vi "Get Grouped Channel Settings.vi"(9 "Type":T2(ring), 10 "Group Name":string, 11 "Group Settings":T3[](array[typedef])) -> (1 "found?":bool, 2 "Channel Settings":T1[](array[typedef]), 3 "Name based Group Settings":T3[](array[typedef]))   [LabVIEW 2026, in "SystemMonitor Engine.lvlib" / "SystemMonitor Engine.lvclass"]
uses:
  SystemMonitor Engine.lvclass
  Shared/GroupSettings.ctl
  Shared/GroupedChannel.ctl
  SystemMonitor Engine.lvclass/SystemMonitor Engine.ctl
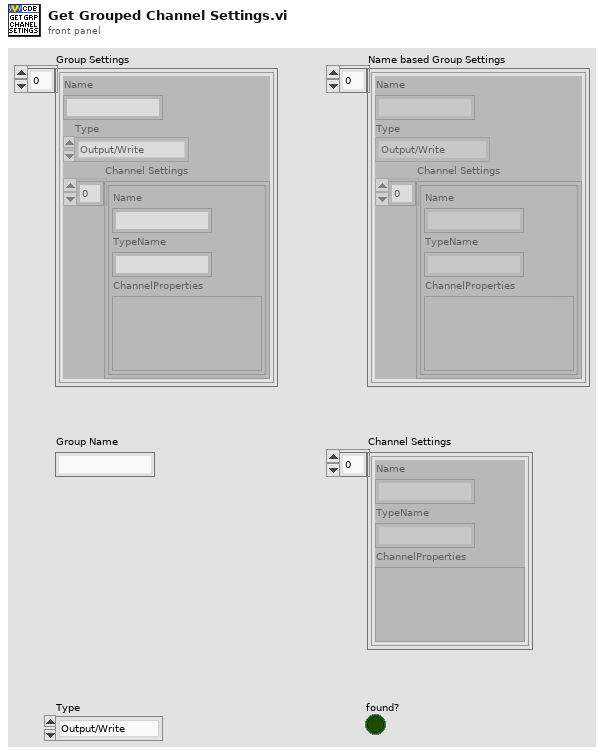
[diagram p1: front panel]
types:
  T1 = typedef "GroupedChannel.ctl" = cluster{"Name":string, "TypeName":string, "ChannelProperties":variant}
  T2 = enum16{"Output/Write", "Input/Read", "Input/ReadWrite"}
  T3 = typedef "GroupSettings.ctl" = cluster{"Name":string, "Type":enum16{"Output/Write", "Input/Read", "Input/ReadWrite"}, "Channel Settings":T1[]}
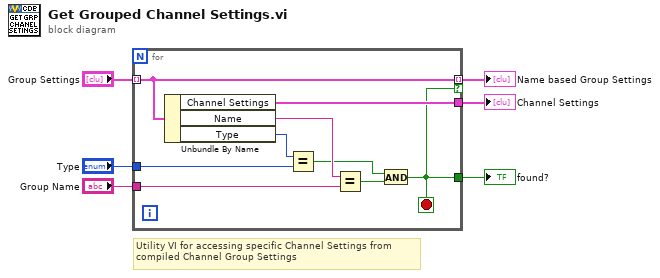
[diagram p0: block diagram]
diagram:
  # "Utility VI for accessing specific Channel Settings from \ncompiled Channel Group Settings"
  n1 = for {
    tunnel: "Group Settings" -> [w9] mode=indexing
    tunnel: "Group Name" -> [w14]
    tunnel: [w7] -> w4
    tunnel: [w9] -> w3 mode=indexing if=w7
    tunnel: "Type" -> [w12]
    tunnel: [w8] -> w1
    stop <- w7 stop-if-true
    n2 = Unbundle By Name(w9) -> ("Channel Settings"=w8:T1[], "Name"=w15:string, "Type"=w13:T2)
    n3 = Equal?(x=w13, y=w12) -> (x = y?=w10:bool)
    n4 = Equal?(x=w15, y=w14) -> (x = y?=w11:bool)
    n5 = And(x=w10, y=w11) -> (x .and. y?=w7:bool)
  }
  "found?" <- w4
  "Name based Group Settings" <- w3
  "Channel Settings" <- w1
